vi "Read Test Case object from front panel control.vi"(8 "error in (no error)":errorcluster, 11 "Test Case in":refnum<class "LUnit Test Case V2.lvclass">) -> (0 "error out":errorcluster, 3 "Test Case out":refnum<class "LUnit Test Case V2.lvclass">)   [LabVIEW 2020, in "LUnit Test Case V2.lvclass"]
uses:
  LUnit Test Case V2.lvclass
  LUnit Test Case V2.lvclass/LUnit Test Case V2.ctl
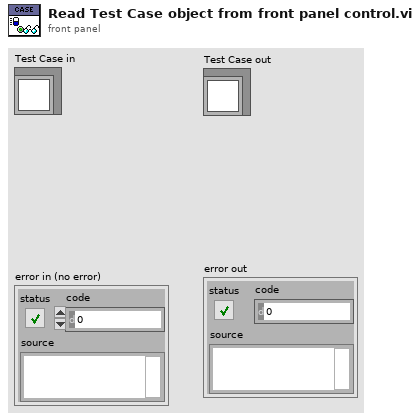
[diagram p1: front panel]
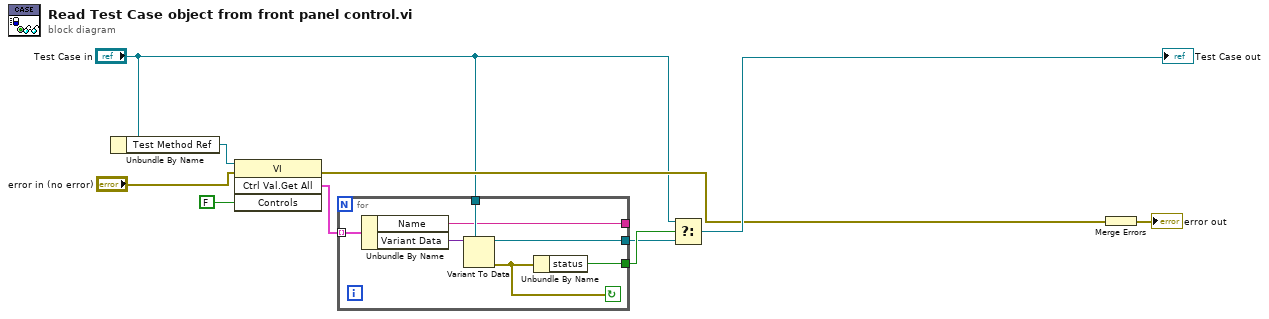
[diagram p0: block diagram]
diagram:
  n1 = Unbundle By Name("Test Case in") -> ("Test Method Ref"=w1:refnum<vi>)
  n2 = invoke on="Invoke Node" class="VI" method="Ctrl Val.Get All"(reference=w1, error in="error in (no error)", "Controls"=FALSE) -> (error out=w7:errorcluster, "Get All Control Values Variant"=w3:cluster{"Name":string, "Variant Data":variant}[])  [unwired: 1 in, 2 out]
  n3 = for {
    tunnel: w3 -> [w17] mode=indexing
    tunnel: "Test Case in" -> [w15]
    tunnel: [w14] -> _
    tunnel: [w12] -> w5
    tunnel: [w11] -> w4
    stop <- w13 continue-if-true
    n4 = Unbundle By Name(w17) -> ("Name"=w14:string, "Variant Data"=w16:variant)
    n5 = Variant To Data(type=w15, Variant=w16) -> (data=w11:refnum<class "LUnit Test Case V2.lvclass">, error out=w13:errorcluster)  [unwired: 1 in]
    n6 = Unbundle By Name(w13) -> ("status"=w12:bool)
  }
  n7 = Select(t="Test Case in", s=w5, f=w4) -> (s? t:f=→"Test Case out":refnum<class "LUnit Test Case V2.lvclass">)
  n8 = Merge Errors(w7) -> (→"error out":errorcluster)
